vi "RTM - Add Diagnostic Channels.vi"(8 "error in (no error)":errorcluster, 11 "Node Ptr":u64 format="%.0x") -> (0 "error out":errorcluster)   [LabVIEW 2016, in "UDP-Custom-Device System Explorer.lvlib"]
uses:
  UDP-Custom-Device System Explorer.lvlib
  Shared/Constants.vi
  <vilib>/NI VeriStand/Custom Device API/Custom Device API.lvlib
  Shared/UDP-Custom-Device Shared.lvlib
  <vilib>/NI Veristand/Custom Device API/Custom Device Channel Type.ctl
  <vilib>/NI Veristand/Custom Device API/Custom Device Channel.ctl
  <vilib>/NI Veristand/Custom Device API/Set Item Property (Boolean).vi
panel:
  in  "Tag":string
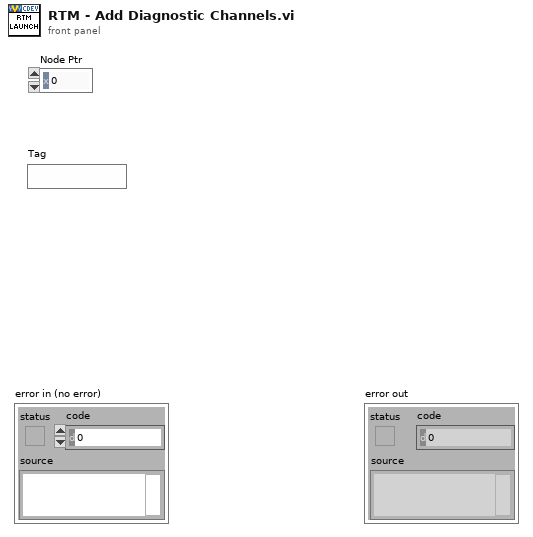
[diagram p1: front panel]
types:
  T1 = typedef "Custom Device API.lvlib/Custom Device Channel.ctl" = cluster{"Type":T2, "Units":string, "Default Value":dbl, "Faultable":bool, "Scalable":bool}
  T2 = typedef "Custom Device API.lvlib/Custom Device Channel Type.ctl" = enum16{"Input", "Output"}
  T3 = typedef "Custom Device API.lvlib/Custom Device Item Ref.ctl" = u64
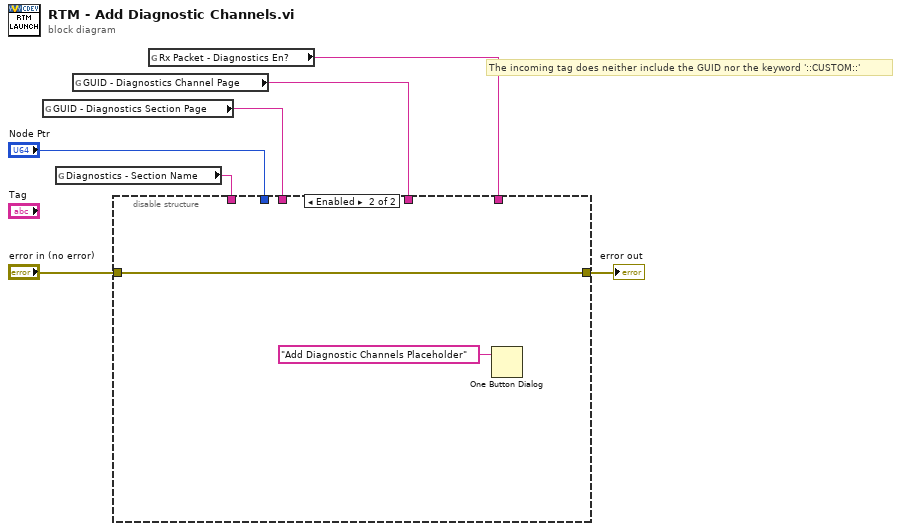
[diagram p0: block diagram]
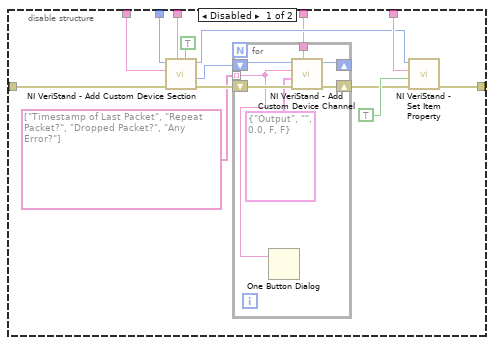
[diagram p2: hidden frame]
diagram:
  # "The incoming tag does neither include the GUID nor the keyword '::CUSTOM::'"
  n1 = global read "Constants.vi" "GUID - Diagnostics Section Page"() -> (w4:string)
  n2 = global read "Constants.vi" "Diagnostics - Section Name"() -> (w5:string)
  n3 = global read "Constants.vi" "GUID - Diagnostics Channel Page"() -> (w1:string)
  n4 = global read "Constants.vi" "Rx Packet - Diagnostics En?"() -> (w2:string)
  n5 = disable-structure shown="Enabled" {
    disable-tunnel: "error in (no error)" -> [w21 w30]
    disable-tunnel: "Node Ptr" -> [w19 _]
    disable-tunnel: w5 -> [w18 _]
    disable-tunnel: w4 -> [w17 _]
    disable-tunnel: [w15 w30] -> w3
    disable-tunnel: w2 -> [w14 _]
    disable-tunnel: w1 -> [w10 _]
    frame Disabled {
      n6 = call <vilib>:"NI VeriStand - Add Custom Device Section.vi"("Highlight? (F)"=TRUE, "GUID (Default Section)"=w17, "error in (no error)"=w21, "Section Name"=w18, "Parent Ref in"=w19) -> ("error out"=w20:errorcluster, "Section Ptr"=w9:T3, "Parent Ref out"=w13:T3)  [unwired: 3 in, 1 out]
      n7 = for {
        tunnel: w10 -> [w26]
        shift-right: [w27] -> w11
        shift-left: w20 -> [w28]
        tunnel: string[] ["Timestamp of Last Packet", "Repeat Packet?", "Dropped Packet?", "Any Error?"] -> [w22] mode=indexing
        shift-right: [w23] -> _
        shift-left: w9 -> [w25]
        n8 = One Button Dialog(message=w22) -> ()  [unwired: 1 in, 1 out]
        n9 = call <vilib>:"NI VeriStand - Add Custom Device Channel.vi"("GUID (Default Channel)"=w26, "error in (no error)"=w28, "Channel"=T1 {"Type"=enum."Output", "Units"="", "Default Value"=0.0, "Faultable"=FALSE, "Scalable"=FALSE}, "Channel Name"=w22, "Parent Ref in"=w25) -> ("error out"=w27:errorcluster, "Parent Ref out"=w23:T3)  [unwired: 3 in, 2 out]
      }
      n10 = call-poly <vilib>:"NI VeriStand - Set Item Property.vi"("error in (no error)"=w11, "Value"=TRUE, "Property Name"=w14, "Item Ref in"=w13) -> ("error out"=w15:errorcluster)  [unwired: 5 in, 2 out]
    }
    frame Enabled {
      n11 = One Button Dialog(message="Add Diagnostic Channels Placeholder") -> ()  [unwired: 1 in, 1 out]
    }
  }
  "error out" <- w3
